vi "Do.vi"(8 "error in (no error)":errorcluster, 9 "CommandQueueIn":refnum<queue>, 10 "DataNotifierIn":refnum<notifier>, 11 "RootCommand in":refnum<class "RootCommand.lvclass">) -> (0 "error out":errorcluster, 1 "ExitFlag":bool, 2 "DataNotifierOut":refnum<notifier>, 3 "RootCommand out":refnum<class "RootCommand.lvclass">)   [LabVIEW 2013, in "RootCommand.lvclass"]
uses:
  RootCommand.lvclass
  SystemData.lvclass/SystemData.lvclass
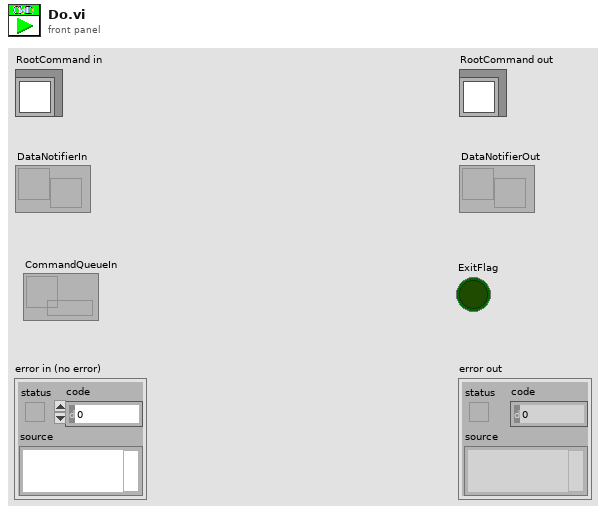
[diagram p1: front panel]
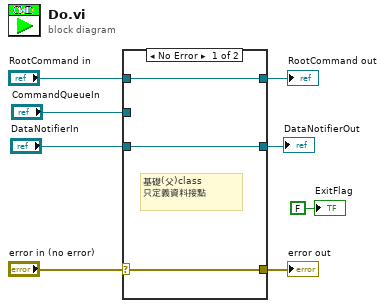
[diagram p0: block diagram]
diagram:
  n1 = case shown="No Error" "error in (no error)" {
    selector: "error in (no error)" -> [w9 w14]
    tunnel: [w9 w14] -> w7
    tunnel: [w11 w13] -> w5
    tunnel: "RootCommand in" -> [w11 w13]
    tunnel: "DataNotifierIn" -> [w10 w12]
    tunnel: [w10 w12] -> w3
    tunnel: "CommandQueueIn" -> [_ _]
    frame No Error {
      # "基礎(父)class\n只定義資料接點"
    }
    frame Error {
    }
  }
  "error out" <- w7
  "RootCommand out" <- w5
  "DataNotifierOut" <- w3
  "ExitFlag" <- FALSE ("ExitFlag")
